vi "TPNT_Args2TP.vi"(9 "key":string, 10 "value":string, 11 "TP_IN":T1={"name"="", "type"="", "algor"=[], "update_rate"=0.0, "Limits"={"Alarm Type"="", "Lower "=0.0, "Upper"=0.0, "Nominal"=0.0, "outrange"=FALSE, "Check"=TRUE, "latch"=FALSE, "level"=""}, "Samples"={"samples"=0, "counter"=0, "Values"=[], "Current Value"="", "filter"="", "precision"=2}, "next_update"=0, "Status"="", "monitor"=TRUE, "error"=FALSE, "Log"={"log"=FALSE, "file"=path "", "type"="", "format"="", "updaterate"=0.0, "nex_update"=0, "mode"=""}, "permissions"="", "ID"=""} {"Log"."updaterate" format="%.2f"; "Samples"."Values" format="%.2f"; "Samples"."samples" min=1 step=1; "Limits"."Nominal" format="%.2f"; "Limits"."Upper" format="%.2f"; "Limits"."Lower" format="%.2f"; "update_rate" format="%.2f"}) -> (3 "TP_OUT":T1={"name"="", "type"="", "algor"=[], "update_rate"=0.0, "Limits"={"Alarm Type"="", "Lower "=0.0, "Upper"=0.0, "Nominal"=0.0, "outrange"=FALSE, "Check"=TRUE, "latch"=FALSE, "level"=""}, "Samples"={"samples"=0, "counter"=0, "Values"=[], "Current Value"="", "filter"="", "precision"=2}, "next_update"=0, "Status"="", "monitor"=TRUE, "error"=FALSE, "Log"={"log"=FALSE, "file"=path "", "type"="", "format"="", "updaterate"=0.0, "nex_update"=0, "mode"=""}, "permissions"="", "ID"=""} {"Log"."updaterate" format="%.2f"; "Samples"."Values" format="%.2f"; "Samples"."samples" min=1 step=1; "Limits"."Nominal" format="%.2f"; "Limits"."Upper" format="%.2f"; "Limits"."Lower" format="%.2f"; "update_rate" format="%.2f"})   [LabVIEW 2016]
uses:
  TPNT_TP.ctl
  TPNT_Limits.ctl
  TPNT_Samples.ctl
  TPNT_Log.ctl
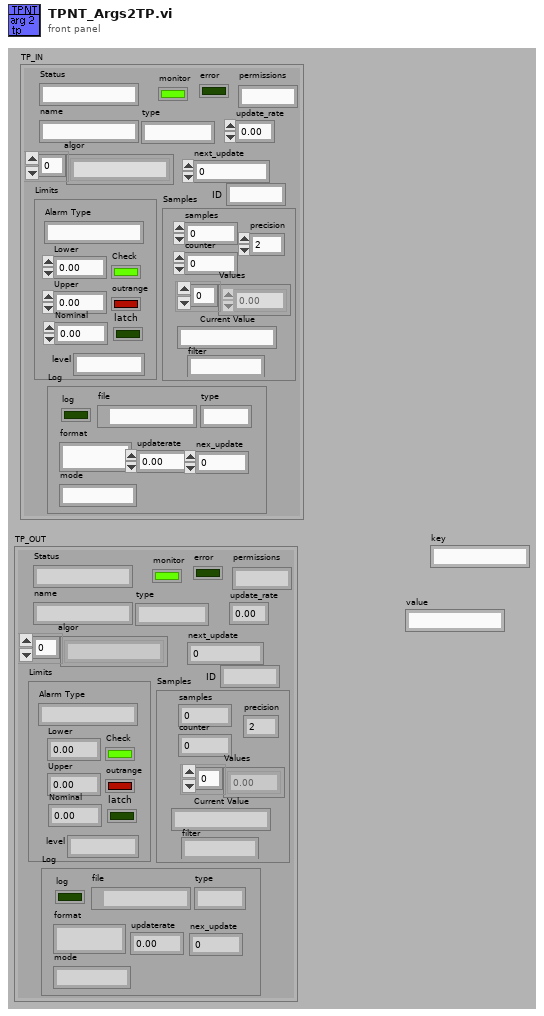
[diagram p1: front panel]
types:
  T1 = typedef "TPNT_TP.ctl" = cluster{"name":string, "type":string, "algor":string[], "update_rate":sgl, "Limits":T2, "Samples":T3, "next_update":u32, "Status":string, "monitor":bool, "error":bool, "Log":T4, "permissions":string, "ID":string}
  T2 = typedef "TPNT_Limits.ctl" = cluster{"Alarm Type":string, "Lower ":dbl, "Upper":dbl, "Nominal":dbl, "outrange":bool, "Check":bool, "latch":bool, "level":string}
  T3 = typedef "TPNT_Samples.ctl" = cluster{"samples":i32, "counter":i32, "Values":dbl[], "Current Value":string, "filter":string, "precision":u8}
  T4 = typedef "TPNT_Log.ctl" = cluster{"log":bool, "file":path, "type":string, "format":string, "updaterate":dbl, "nex_update":u32, "mode":string}
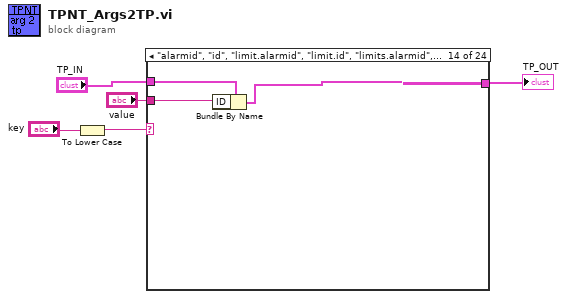
[diagram p0: block diagram]
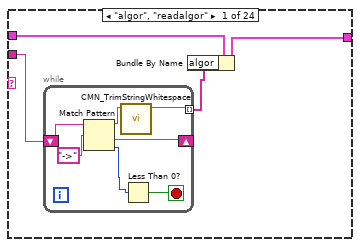
[diagram p2: hidden frame]
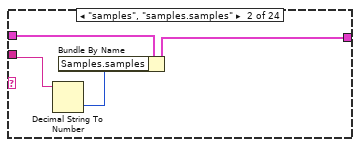
[diagram p3: hidden frame]
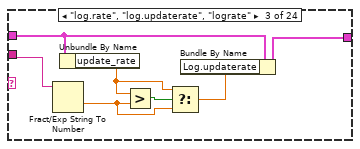
[diagram p4: hidden frame]
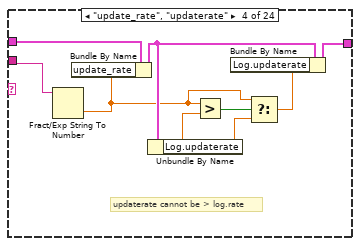
[diagram p5: hidden frame]
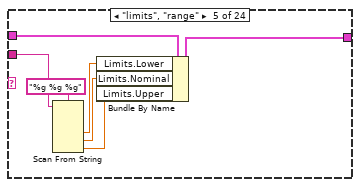
[diagram p6: hidden frame]
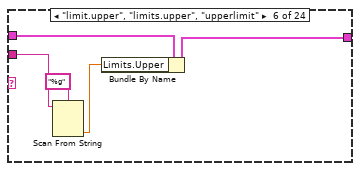
[diagram p7: hidden frame]
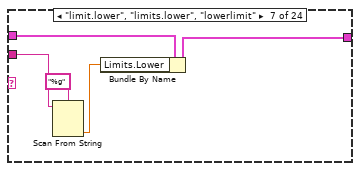
[diagram p8: hidden frame]
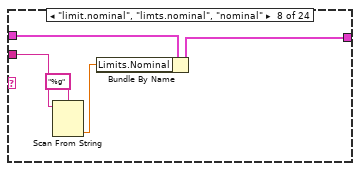
[diagram p9: hidden frame]
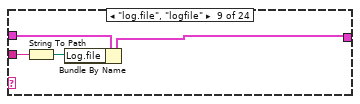
[diagram p10: hidden frame]
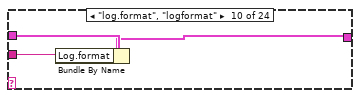
[diagram p11: hidden frame]
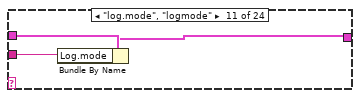
[diagram p12: hidden frame]
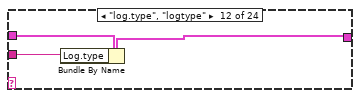
[diagram p13: hidden frame]
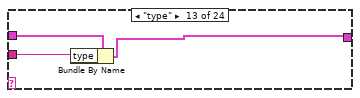
[diagram p14: hidden frame]
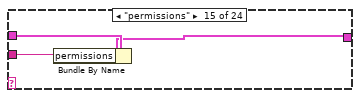
[diagram p15: hidden frame]
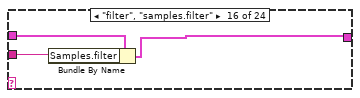
[diagram p16: hidden frame]
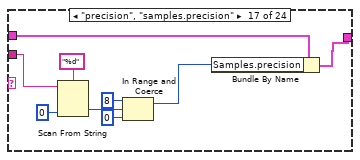
[diagram p17: hidden frame]
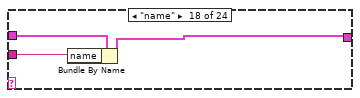
[diagram p18: hidden frame]
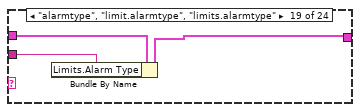
[diagram p19: hidden frame]
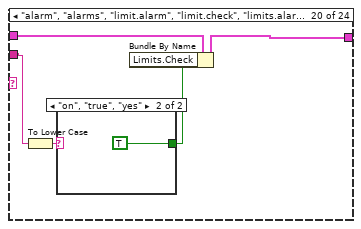
[diagram p20: hidden frame]
diagram:
  n1 = To Lower Case(string="key") -> (all lower case string=w1:string)
  n2 = case shown="\"alarmid\", \"id\", \"limit.alarmid\", \"limit.id\", \"limits.alarmid\", \"limits.id\"" w1 {
    tunnel: "TP_IN" -> [w9 w20 w25 w35 w42 w47 w52 w57 w61 w64 w67 w70 w73 w76 w79 w81 w91 w94 w96 w102 w109 w116 w123 w126]
    tunnel: "value" -> [w7 w18 w26 w34 w40 w45 w50 w55 w59 w62 w65 w68 w71 w74 w77 w82 w89 w92 w97 w98 w105 w113 w119 _]
    tunnel: [w8 w19 w27 w31 w41 w46 w51 w56 w60 w63 w66 w69 w72 w75 w78 w80 w90 w93 w95 w101 w108 w115 w122 w126] -> w4
    frame "algor", "readalgor" {
      n3 = while {
        tunnel: [w10] -> w6 mode=indexing
        shift-right: [w13] -> _
        shift-left: w7 -> [w12]
        stop <- w14 stop-if-true
        n4 = Match Pattern(string=w12, regular expression="->") -> (before substring=w11:string, after substring=w13:string, offset past match=w15:i32)  [unwired: 2 out]
        n5 = call "CMN_TrimStringWhitespace.vi"("string"=w11) -> ("trimmed string"=w10:string)  [unwired: 1 in, 8 out]
        n6 = Less Than 0?(x=w15) -> (x < 0?=w14:bool)
      }
      n7 = Bundle By Name(cluster=w9, "algor"=w6) -> (w8:T1)
    }
    frame "samples", "samples.samples" {
      n8 = Decimal String To Number(string=w18) -> (number=w17:i32)  [unwired: 3 out]
      n9 = Bundle By Name(cluster=w20, "Samples.samples"=w17) -> (w19:T1)
    }
    frame "log.rate", "log.updaterate", "lograte" {
      n10 = Fract/Exp String To Number(string=w26) -> (number=w22:dbl)  [unwired: 4 out]
      n11 = Unbundle By Name(w25) -> ("update_rate"=w23:sgl)
      n12 = Greater?(x=w23, y=w22) -> (0:w24:bool)
      n13 = Select(t=w23, s=w24, f=w22) -> (s? t:f=w21:dbl)
      n14 = Bundle By Name(cluster=w25, "Log.updaterate"=w21) -> (w27:T1)
    }
    frame "update_rate", "updaterate" {
      # "updaterate cannot be > log.rate"
      n15 = Fract/Exp String To Number(string=w34) -> (number=w30:dbl)  [unwired: 4 out]
      n16 = Bundle By Name(cluster=w35, "update_rate"=w30) -> (w32:T1)
      n17 = Unbundle By Name(w32) -> ("Log.updaterate"=w29:dbl)
      n18 = Greater?(x=w30, y=w29) -> (0:w33:bool)
      n19 = Select(t=w30, s=w33, f=w29) -> (s? t:f=w28:dbl)
      n20 = Bundle By Name(cluster=w32, "Log.updaterate"=w28) -> (w31:T1)
    }
    frame "limits", "range" {
      n21 = Scan From String(format string="%g %g %g", input string=w40) -> (output 1=w38:dbl, output 2=w36:dbl, output 3=w37:dbl)  [unwired: 2 in, 6 out]
      n22 = Bundle By Name(cluster=w42, "Limits.Lower"=w38, "Limits.Nominal"=w36, "Limits.Upper"=w37) -> (w41:T1)
    }
    frame "limit.upper", "limits.upper", "upperlimit" {
      n23 = Scan From String(format string="%g", input string=w45) -> (output 1=w43:dbl)  [unwired: 2 in, 4 out]
      n24 = Bundle By Name(cluster=w47, "Limits.Upper"=w43) -> (w46:T1)
    }
    frame "limit.lower", "limits.lower", "lowerlimit" {
      n25 = Scan From String(format string="%g", input string=w50) -> (output 1=w48:dbl)  [unwired: 2 in, 4 out]
      n26 = Bundle By Name(cluster=w52, "Limits.Lower"=w48) -> (w51:T1)
    }
    frame "limit.nominal", "limts.nominal", "nominal" {
      n27 = Scan From String(format string="%g", input string=w55) -> (output 1=w53:dbl)  [unwired: 2 in, 4 out]
      n28 = Bundle By Name(cluster=w57, "Limits.Nominal"=w53) -> (w56:T1)
    }
    frame "log.file", "logfile" {
      n29 = String To Path(string=w59) -> (path=w58:path)
      n30 = Bundle By Name(cluster=w61, "Log.file"=w58) -> (w60:T1)
    }
    frame "log.format", "logformat" {
      n31 = Bundle By Name(cluster=w64, "Log.format"=w62) -> (w63:T1)
    }
    frame "log.mode", "logmode" {
      n32 = Bundle By Name(cluster=w67, "Log.mode"=w65) -> (w66:T1)
    }
    frame "log.type", "logtype" {
      n33 = Bundle By Name(cluster=w70, "Log.type"=w68) -> (w69:T1)
    }
    frame "type" {
      n34 = Bundle By Name(cluster=w73, "type"=w71) -> (w72:T1)
    }
    frame "alarmid", "id", "limit.alarmid", "limit.id", "limits.alarmid", "limits.id" {
      n35 = Bundle By Name(cluster=w76, "ID"=w74) -> (w75:T1)
    }
    frame "permissions" {
      n36 = Bundle By Name(cluster=w79, "permissions"=w77) -> (w78:T1)
    }
    frame "filter", "samples.filter" {
      n37 = Bundle By Name(cluster=w81, "Samples.filter"=w82) -> (w80:T1)
    }
    frame "precision", "samples.precision" {
      n38 = Scan From String(format string="%d", input string=w89, default 1=u8 0 ("default value 1")) -> (output 1=w87:u8)  [unwired: 2 in, 3 out]
      n39 = In Range and Coerce(upper limit=u8 8, x=w87, lower limit=u8 0) -> (coerced(x)=w84:u8)  [unwired: 1 out]
      n40 = Bundle By Name(cluster=w91, "Samples.precision"=w84) -> (w90:T1)
    }
    frame "name" {
      n41 = Bundle By Name(cluster=w94, "name"=w92) -> (w93:T1)
    }
    frame "alarmtype", "limit.alarmtype", "limits.alarmtype" {
      n42 = Bundle By Name(cluster=w96, "Limits.Alarm Type"=w97) -> (w95:T1)
    }
    frame "alarm", "alarms", "limit.alarm", "limit.check", "limits.alarm" {
      n43 = To Lower Case(string=w98) -> (all lower case string=w99:string)
      n44 = case shown="\"on\", \"true\", \"yes\"" w99 {
        tunnel: [FALSE TRUE] -> w100
        frame Default {
        }
        frame "on", "true", "yes" {
        }
      }
      n45 = Bundle By Name(cluster=w102, "Limits.Check"=w100) -> (w101:T1)
    }
    frame "alarmlatch", "limit.alarmlatch", "limit.latch", "limits.alarmlatch" {
      n46 = To Lower Case(string=w105) -> (all lower case string=w106:string)
      n47 = case shown="\"on\", \"true\", \"yes\"" w106 {
        tunnel: [FALSE TRUE] -> w107
        frame Default {
        }
        frame "on", "true", "yes" {
        }
      }
      n48 = Bundle By Name(cluster=w109, "Limits.latch"=w107) -> (w108:T1)
    }
    frame "monitor", "monitoring" {
      n49 = To Lower Case(string=w113) -> (all lower case string=w114:string)
      n50 = case shown="\"on\", \"true\", \"yes\"" w114 {
        tunnel: [FALSE TRUE] -> w112
        frame Default {
        }
        frame "on", "true", "yes" {
        }
      }
      n51 = Bundle By Name(cluster=w116, "monitor"=w112) -> (w115:T1)
    }
    frame "log", "log.log", "logging" {
      n52 = To Lower Case(string=w119) -> (all lower case string=w121:string)
      n53 = case shown="\"on\", \"true\", \"yes\"" w121 {
        tunnel: [FALSE TRUE] -> w120
        frame Default {
        }
        frame "on", "true", "yes" {
        }
      }
      n54 = Bundle By Name(cluster=w123, "Log.log"=w120) -> (w122:T1)
    }
    frame Default {
    }
  }
  "TP_OUT" <- w4
